vi "CLSUIP_WireUpIndexArray.vi"(8 "error in (no error)":errorcluster, 10 "Unwired Terminals":refnum<vi>[](array[refnum]), 11 "Index Array Ref":refnum<vi>) -> (0 "error out":errorcluster, 3 "Index Array Ref out":refnum<vi>)   [LabVIEW 2021, in "MemberVICreation.lvlib"]
uses:
  <resource>/Framework/Providers/LVClassLibrary/NewAccessors/MemberVICreation.lvlib
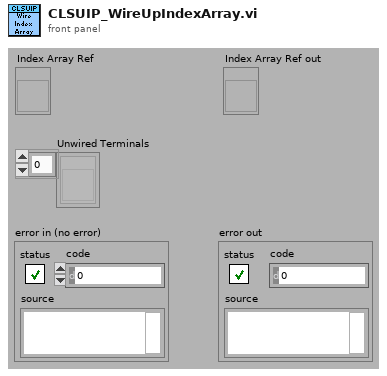
[diagram p1: front panel]
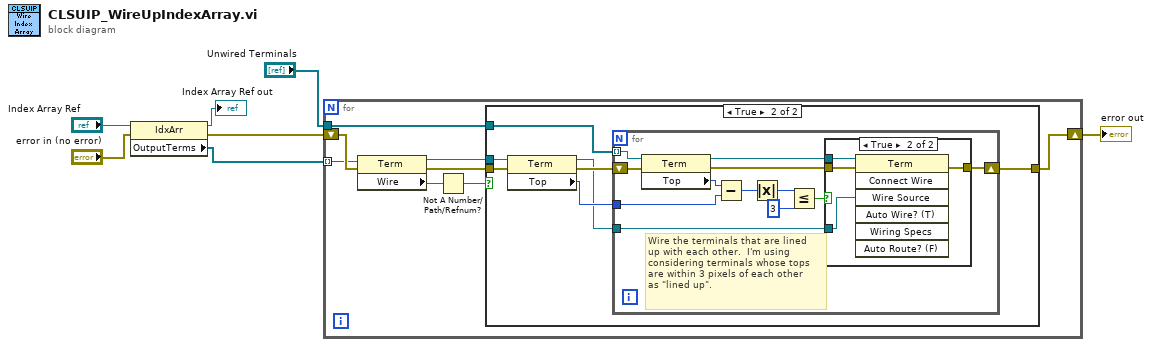
[diagram p0: block diagram]
diagram:
  n1 = property class="IdxArr"(reference="Index Array Ref", error in="error in (no error)") -> (reference out=→"Index Array Ref out":refnum<vi>, error out=w2:errorcluster, "OutputTerms"=w3:refnum<vi>[])
  n2 = for {
    tunnel: "Unwired Terminals" -> [w11]
    shift-right: [w8] -> w7
    shift-left: w2 -> [w15]
    tunnel: w3 -> [w14] mode=indexing
    n3 = property class="Term"(reference=w14, error in=w15) -> (reference out=w10:refnum<vi>, error out=w9:errorcluster, "Wire"=w13:refnum<vi>)
    n4 = Not A Number/Path/Refnum?(number/path/refnum=w13) -> (NaN/Path/Refnum?=w12:bool)
    n5 = case shown="True" w12 {
      tunnel: w11 -> [_ w20]
      tunnel: w10 -> [_ w23]
      tunnel: w9 -> [w16 w22]
      tunnel: [w16 w17] -> w8
      frame False {
        # "If it's already wired, we don't have to worry about it."
      }
      frame True {
        n6 = property class="Term"(reference=w23, error in=w22) -> (reference out=w18:refnum<vi>, error out=w19:errorcluster, "Top"=w21:i32)
        n7 = for {
          tunnel: w21 -> [w32]
          tunnel: w20 -> [w35] mode=indexing
          shift-right: [w24] -> w17
          shift-left: w19 -> [w34]
          tunnel: w18 -> [w25]
          # "Wire the terminals that are lined\nup with each other.  I'm using\nconsidering terminals whose tops\nare within 3 pixels of each other\nas \"lined up\"."
          n8 = property class="Term"(reference=w35, error in=w34) -> (reference out=w26:refnum<vi>, error out=w27:errorcluster, "Top"=w33:i32)
          n9 = Subtract(x=w33, y=w32) -> (x-y=w31:i32)
          n10 = Absolute Value(x=w31) -> (abs(x)=w30:i32)
          n11 = Less Or Equal?(x=w30, y=3) -> (x <= y?=w28:bool)
          n12 = case shown="True" w28 {
            tunnel: w27 -> [w36 w40]
            tunnel: w26 -> [_ w39]
            tunnel: w25 -> [_ w38]
            tunnel: [w36 w37] -> w24
            frame False {
            }
            frame True {
              n13 = invoke class="Term" method="Connect Wire"(reference=w39, error in=w40, "Wire Source"=w38) -> (error out=w37:errorcluster)  [unwired: 4 in, 6 out]
            }
          }
        }
      }
    }
  }
  "error out" <- w7
